vi "Distance State Logic.vi"(9 "Back":bool, 10 "Mid":bool, 11 "Front":bool) -> (3 "Shooting State":T1)   [LabVIEW 2019, in "Robot.lvlib" / "Panzer.lvclass"]
uses:
  Panzer.lvclass
  PowerCellHandler/Controls/Shooting Position.ctl
  <vilib>/Rock Robotics/Network Tables/NT Write String.vi
  PowerCellHandler/Power Cell Handler.lvclass
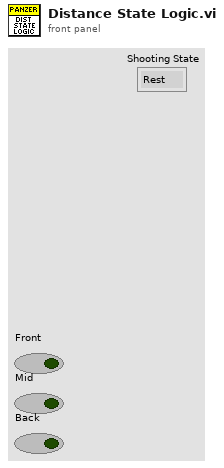
[diagram p1: front panel]
types:
  T1 = typedef "Power Cell Handler.lvlib/Power Cell Handler.lvclass/Shooting Position.ctl" = enum16{"Rest", "Front", "Middle", "Back"}
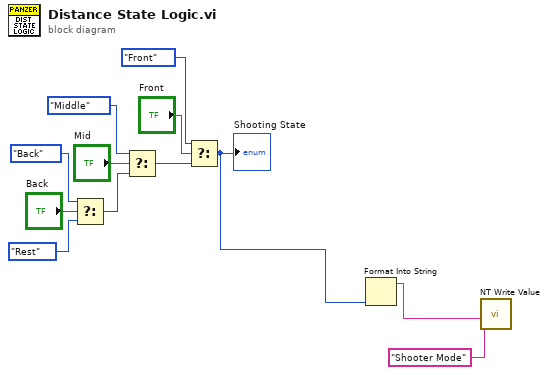
[diagram p0: block diagram]
diagram:
  n1 = Select(t=Shooting_Position."Back" ("Shooting Position"), s="Back", f=Shooting_Position."Rest" ("Shooting Position")) -> (s? t:f=w12:T1)
  n2 = Select(t=Shooting_Position."Middle" ("Shooting Position"), s="Mid", f=w12) -> (s? t:f=w11:T1)
  n3 = Select(t=Shooting_Position."Front" ("Shooting Position"), s="Front", f=w11) -> (s? t:f=w3:T1)
  "Shooting State" <- w3
  n4 = Format Into String(w3) -> (resulting string=w2:string)  [unwired: 3 in, 1 out]
  n5 = call-poly <vilib>:"NT Write Value.vi"("String"=w2, "Name"="Shooter Mode") -> ()  [unwired: 9 in, 1 out]
